vi "HEWH Program Type.vi"(11 "Program Names":T1) -> (2 "Test_Type:":string(combo)="Stand Override", 3 "Program Type":string)   [LabVIEW 2016]
uses:
  Type Definitions/HEWH Program Names.ctl
panel:
  out "Numeric":i32
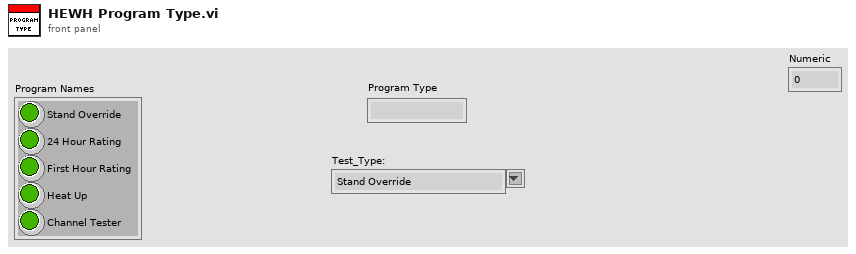
[diagram p1: front panel]
types:
  T1 = typedef "HEWH Program Names.ctl" = cluster{"Stand Override":bool, "24 Hour Rating":bool, "First Hour Rating":bool, "Heat Up":bool, "Channel Tester":bool}
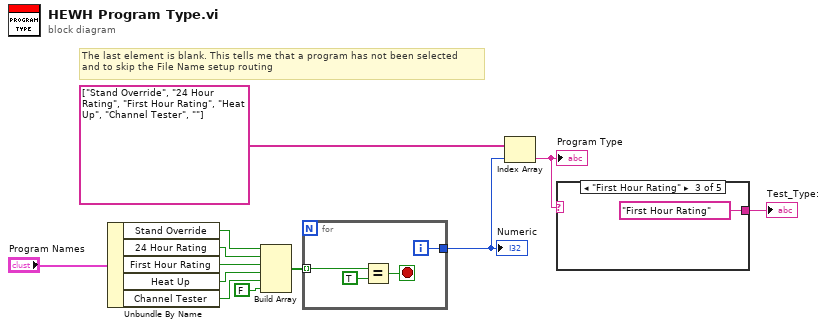
[diagram p0: block diagram]
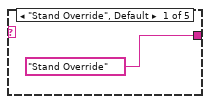
[diagram p2: hidden frame]
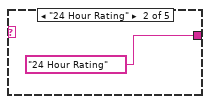
[diagram p3: hidden frame]
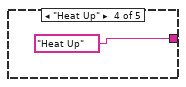
[diagram p4: hidden frame]
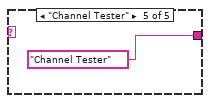
[diagram p5: hidden frame]
diagram:
  # "The last element is blank. This tells me that a program has not been selected\nand to skip the File Name setup routing"
  n1 = Unbundle By Name("Program Names") -> ("Stand Override"=w11:bool, "24 Hour Rating"=w10:bool, "First Hour Rating"=w9:bool, "Heat Up"=w8:bool, "Channel Tester"=w7:bool)
  n2 = Build Array(w11, w10, w9, w8, w7, FALSE) -> (w6:bool[])
  n3 = for {
    tunnel: w6 -> [w16] mode=indexing
    tunnel: [w13] -> w4
    i -> [w13]
    stop <- w14 stop-if-true
    n4 = Equal?(x=w16, y=TRUE) -> (x = y?=w14:bool)
  }
  "Numeric" <- w4
  n5 = Index Array(array=string[] ["Stand Override", "24 Hour Rating", "First Hour Rating", "Heat Up", "Channel Tester", ""], index=w4) -> (element=w2:string)
  "Program Type" <- w2
  n6 = case shown="\"First Hour Rating\"" w2 {
    tunnel: ["Stand Override" ("Test_Type:") "24 Hour Rating" ("Test_Type:") "First Hour Rating" ("Test_Type:") "Heat Up" ("Test_Type:") "Channel Tester" ("Test_Type:")] -> w1
    frame "Stand Override", Default {
    }
    frame "24 Hour Rating" {
    }
    frame "First Hour Rating" {
    }
    frame "Heat Up" {
    }
    frame "Channel Tester" {
    }
  }
  "Test_Type:" <- w1
